vi "Simple AAV.vi"() -> ()   [LabVIEW 2014]
doc: "该VI可用于采集、分析和演示数据。该VI是LabVIEW核心课程I中练习的答案。步骤信息见教材。"
uses:
  Instance           2 18Saved   Simple AAP .vi
  Instance           3 18Saved   Simple AAP .vi
panel:
  out "波形图":dynamicdata(graph)
  out "平均值":dbl
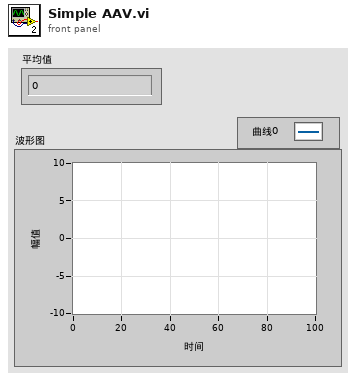
[diagram p1: front panel]
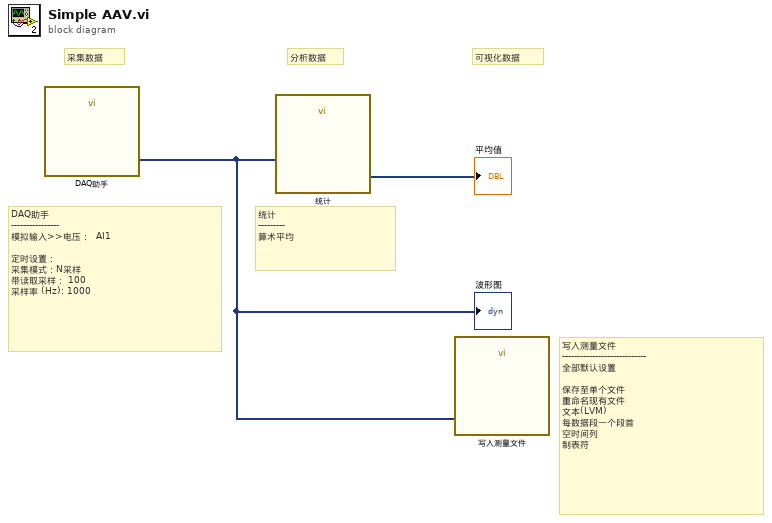
[diagram p0: block diagram]
diagram:
  # "统计\n---------\n算术平均"
  # "写入测量文件\n----------------------------\n全部默认设置\n\n保存至单个文件\n重命名现有文件\n文本(LVM)\n每数据段一个段首\n空时间列\n制表符"
  # "DAQ助手\n----------------\n模拟输入>>电压：  AI1\n\n定时设置：\n采集模式：N采样\n带读取采样： 100\n采样率 (Hz): 1000"
  # "可视化数据"
  # "分析数据"
  # "采集数据"
  n1 = call "DAQ助手"() -> ("data"=w2:dynamicdata)  [unwired: 9 in, 2 out]
  "波形图" <- w2
  n2 = call "统计"("Signals"=w2) -> ("Arithmetic Mean"=→"平均值":dynamicdata)  [unwired: 25 in, 1 out]
  n3 = call "写入测量文件"("Signals"=w2) -> ()  [unwired: 8 in, 3 out]
